vi "Show.vi"(0 "LV MDI in":refnum<class "LV MDI.lvclass">, 7 "Doc Name[]":string[](array[string]), 11 "error in (no error)":errorcluster) -> (4 "LV MDI out":refnum<class "LV MDI.lvclass">, 15 "error out":errorcluster)   [LabVIEW 2016, in "LV MDI.lvclass"]
doc: "Add Documents to the container and display it within the container."
uses:
  LV MDI.lvclass
  LV MDI.lvclass/LV MDI.ctl
  Document/Document.lvclass
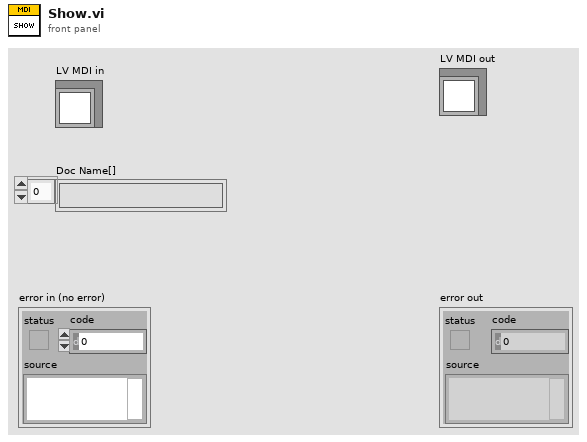
[diagram p1: front panel]
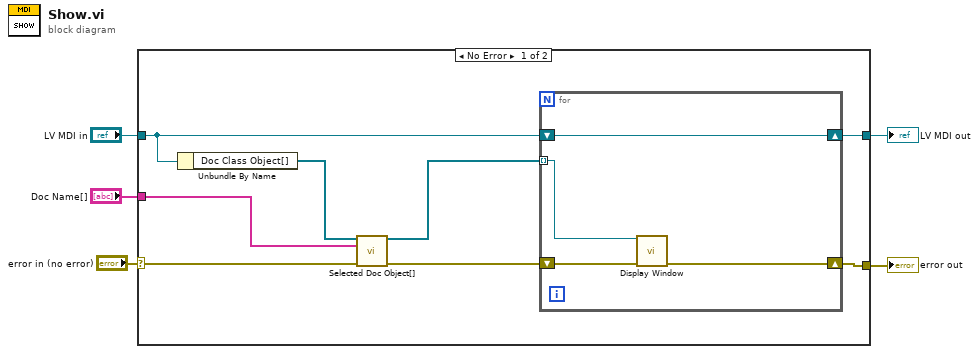
[diagram p0: block diagram]
diagram:
  n1 = case shown="No Error" "error in (no error)" {
    selector: "error in (no error)" -> [w7 w19]
    tunnel: [w13 w19] -> w4
    tunnel: [w11 w18] -> w2
    tunnel: "LV MDI in" -> [w12 w18]
    tunnel: "Doc Name[]" -> [w9 _]
    frame No Error {
      n2 = Unbundle By Name(w12) -> ("Doc Class Object[]"=w10:refnum<class "Document.lvclass">[])
      n3 = call "Selected Doc Object[].vi"("Doc Class Object[]"=w10, "Doc Name[]"=w9, "error in"=w7) -> ("Selected Doc[]"=w8:refnum<class "Document.lvclass">[], "error Out"=w6:errorcluster)  [unwired: 11 in]
      n4 = for {
        shift-right: [w15] -> w13
        shift-left: w6 -> [w16]
        shift-right: [w17] -> w11
        shift-left: w12 -> [w17]
        tunnel: w8 -> [w14] mode=indexing
        n5 = call "Display Window.vi"("Document in"=w14, "error in (no error)"=w16) -> ("error out"=w15:errorcluster)  [unwired: 12 in, 1 out]
      }
    }
    frame Error {
    }
  }
  "error out" <- w4
  "LV MDI out" <- w2
